vi "Query Option List.vi"(8 "error in (no error)":errorcluster, 9 "OptionType (All)":i32(ring) items=["All", "SW Option", "HW Option", "SW Package", "FWA"], 10 "Validity (All)":i32(ring) items=["All", "Valid", "Functional"], 11 "VISA resource name":refnum<visa-resource-name>) -> (0 "error out":errorcluster, 2 "OptionList":string, 3 "VISA resource name out":refnum<visa-resource-name>)   [LabVIEW 2020, in "Rohde&Schwarz CMXP Base.lvlib"]
doc: "Returns a list of installed software options (licenses), hardware options, software packages and firmware applications.\nThe list can be filtered using the described parameters. If filtering results in an empty list, a \"0\" is returned.\nThe meaning of the filter <Validity> depends on the <OptionType> as follows:A software option is valid if there is an active license key for it. The value \"FUNCtional\" is not relevant.A hardware option is functional if the corresponding hardware and all its components can be used (no defect detected). The value \"VALid\" is not relevant.A firmware application is functional if the required hardware, software and license keys are available and functional. The value \"VALid\" is not relevant.For software packages, the filter has no effect.\n\nAttribute:\n-\n\nRemote-control command:\nSYSTem:BASE:OPTion:LIST?"
uses:
  <instrlib>/Rohde&Schwarz CMXP Base/Rohde&Schwarz CMXP Base.lvlib
  <instrlib>/Rohde&Schwarz CMXP Base/Private/rsidr_core.llb/rsidr_core.lvlib
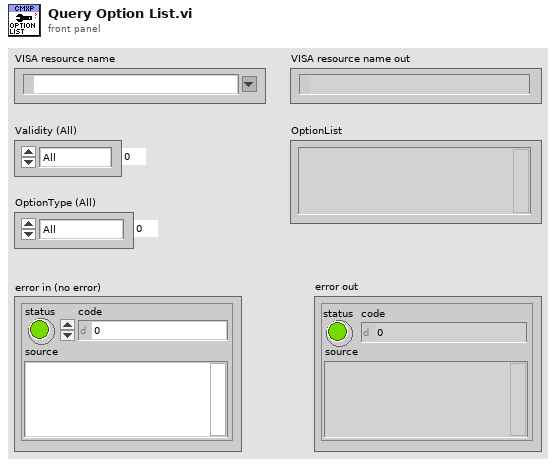
[diagram p1: front panel]
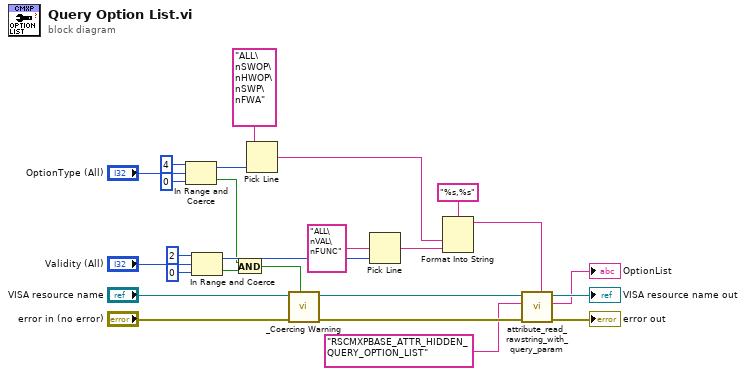
[diagram p0: block diagram]
diagram:
  n1 = In Range and Coerce(upper limit=4, x="OptionType (All)", lower limit=0) -> (coerced(x)=w20:i32, In Range?=w17:bool)
  n2 = In Range and Coerce(upper limit=2, x="Validity (All)", lower limit=0) -> (coerced(x)=w19:i32, In Range?=w18:bool)
  n3 = And(x=w17, y=w18) -> (x .and. y?=w11:bool)
  n4 = Pick Line(multi-line string="ALL\nSWOP\nHWOP\nSWP\nFWA", line index=w20) -> (output string=w1:string)  [unwired: 1 in]
  n5 = call <instrlib>:"_Coercing Warning.vi"("In Range?"=w11, "error in (no error)"="error in (no error)", "VISA resource name"="VISA resource name") -> ("error out"=w8:errorcluster, "VISA resource name out"=w7:refnum<visa-resource-name>)  [unwired: 7 in]
  n6 = Pick Line(multi-line string="ALL\nVAL\nFUNC", line index=w19) -> (output string=w15:string)  [unwired: 1 in]
  n7 = Format Into String(format string="%s,%s", w1, w15) -> (resulting string=w4:string)  [unwired: 2 in, 1 out]
  n8 = call <instrlib>:"attribute_read_rawstring_with_query_param.vi"("Query Parameter (None)"=w4, "error in"=w8, "Attribute ID"="RSCMXPBASE_ATTR_HIDDEN_QUERY_OPTION_LIST", "VISA resource name"=w7) -> ("error out"=→"error out":errorcluster, "RawString out"=→"OptionList":string, "VISA resource name out"=→"VISA resource name out":refnum<visa-resource-name>)  [unwired: 5 in]
